vi "poly_average_ith_value_2d_double_array.vi"(1 "0 indexed? (t)":bool=TRUE, 2 "new array":dbl[][](array[numeric]) format="%#_13g", 3 "old array":dbl[][](array[numeric]) format="%#_13g", 4 "i":i32) -> (7 "average array":dbl[][](array[numeric]))   [LabVIEW 2015, in "_average_tools_polys.lvlib"]
uses:
  _average_tools_polys.lvlib
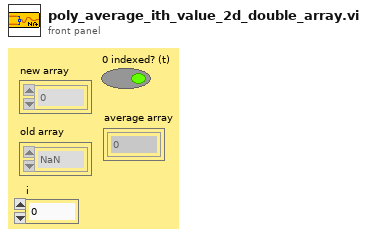
[diagram p1: front panel]
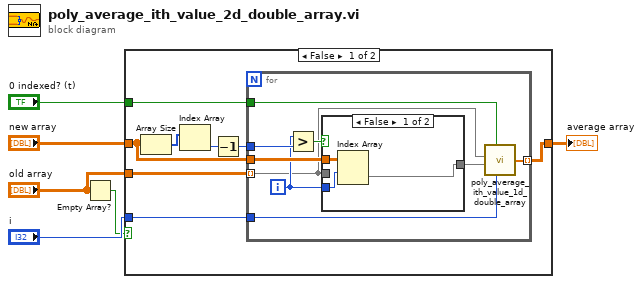
[diagram p0: block diagram]
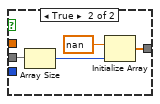
[diagram p2: hidden frame]
diagram:
  n1 = Empty Array?(array="old array") -> (empty?=w1:bool)
  n2 = case shown="False" w1 {
    tunnel: "old array" -> [w14 _]
    tunnel: "new array" -> [w13 w31]
    tunnel: [w11 w31] -> w5
    tunnel: "i" -> [w10 _]
    tunnel: "0 indexed? (t)" -> [w9 _]
    frame False {
      n3 = Array Size(array=w13) -> (size(s)=w8:i32[])
      n4 = Index Array(array=w8) -> (element=w7:i32)  [unwired: 1 in]
      n5 = Decrement(x=w7) -> (x-1=w12:i32)
      n6 = for {
        tunnel: w14 -> [w15] mode=indexing
        tunnel: w13 -> [w23]
        tunnel: w12 -> [w21]
        tunnel: [w16] -> w11 mode=indexing
        tunnel: w10 -> [w17]
        tunnel: w9 -> [w18]
        i -> [w20]
        n7 = Greater?(x=w20, y=w21) -> (0:w22:bool)
        n8 = case shown="False" w22 {
          tunnel: w23 -> [w26 _]
          tunnel: w20 -> [w25 _]
          tunnel: [w24 w27] -> w19
          tunnel: w15 -> [_ w30]
          frame False {
            n9 = Index Array(array=w26, index (row)=w25) -> (element=w24:dbl[])  [unwired: 1 in]
          }
          frame True {
            n10 = Array Size(array=w30) -> (size(s)=w29:i32)
            n11 = Initialize Array(nan ("element"), w29) -> (w27:dbl[])
          }
        }
        n12 = call "poly_average_ith_value_1d_double_array.vi"("0 indexed? (t)"=w18, "new array"=w15, "old array"=w19, "i"=w17) -> ("average array"=w16:dbl[])  [unwired: 4 in]
      }
    }
    frame True {
    }
  }
  "average array" <- w5
